vi "Read Multi U16.vi"(8 "error in (no error)":errorcluster, 9 "Type":u16[](array[numeric]), 10 "Tag":string[](array[string]), 11 "Var Bus in":refnum<class "Omni_Bus.lvclass">) -> (0 "error out":errorcluster, 2 "U16's":u16[](array[numeric]), 3 "Var Bus out":refnum<class "Omni_Bus.lvclass">)   [LabVIEW 2021, in "Omni_Bus.lvclass"]
uses:
  Omni_Bus.lvclass
  <vilib>/TSA/Abstract Data Classes/Abs_Types/U16 Integer/Abs_U16 Integer.lvclass
  Omni_Bus.lvclass/Omni_Bus.ctl
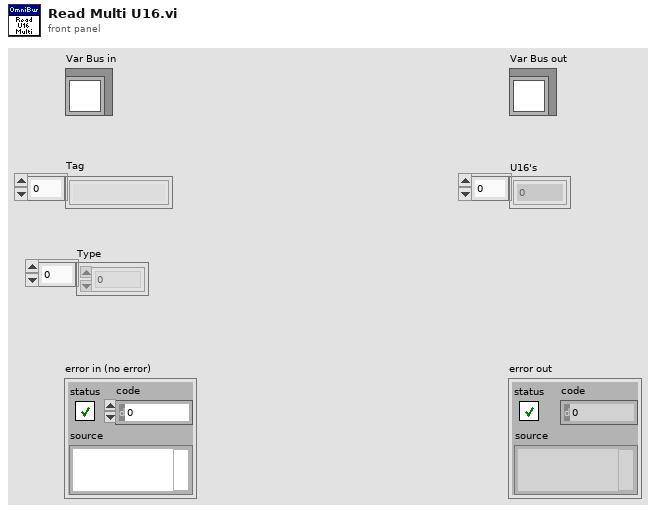
[diagram p1: front panel]
types:
  T1 = typedef "Abs_U16 Integer.lvclass/Type.ctl" = u16
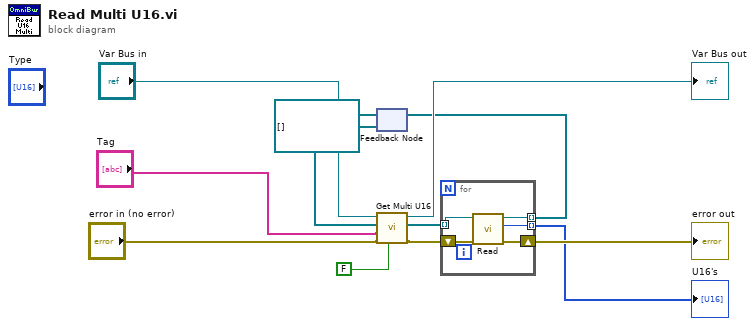
[diagram p0: block diagram]
diagram:
  n1 = feedback #1(refnum<class "Abs_U16 Integer.lvclass">[] []) -> (w3:refnum<class "Abs_U16 Integer.lvclass">[])
  n2 = call-dynamic "Get Multi U16.vi"("Write?"=FALSE, "error in (no error)"="error in (no error)", "Tag"="Tag", "Value Type"=w3, "Var Bus in"="Var Bus in") -> ("error out"=w5:errorcluster, "Value Out"=w4:refnum<class "Abs_U16 Integer.lvclass">[], "Var Bus out"=→"Var Bus out":refnum<class "Omni_Bus.lvclass">)  [unwired: 4 in]
  n3 = for {
    tunnel: [w16] -> w7 mode=indexing
    tunnel: [w15] -> w6 mode=indexing
    tunnel: w4 -> [w13] mode=indexing
    shift-right: [w17] -> w11
    shift-left: w5 -> [w14]
    n4 = call-dynamic "Read.vi"("error in (no error)"=w14, "Double Float.lvclass_340760 in"=w13) -> ("error out"=w17:errorcluster, "Value"=w16:T1, "Double Float.lvclass_340760 out"=w15:refnum<class "Abs_U16 Integer.lvclass">)  [unwired: 7 in]
  }
  "error out" <- w11
  "U16's" <- w7
  n5 = feedback-in #1(w6) -> ()
